vi "Search_Model.vi"(7 "LabVIEW Web Service Request":refnum<class "Web Request.lvclass">) -> (3 "html response":string)   [LabVIEW 2016]
uses:
  <vilib>/wsapi/Web Request.lvclass
  Device Info.ctl
  Inventory FGV Command.ctl
panel:
  # "Use the Web Service Request input terminal to call the VIs on the Web Services palette. Do not remove it from the connector pane unless you don't need access to the palette."
  # "Each additional control wired to the connector pane will be available as an input in the URL. To include an indicator in terminal-mode output (the default setting), it must also be wired to the connector pane."
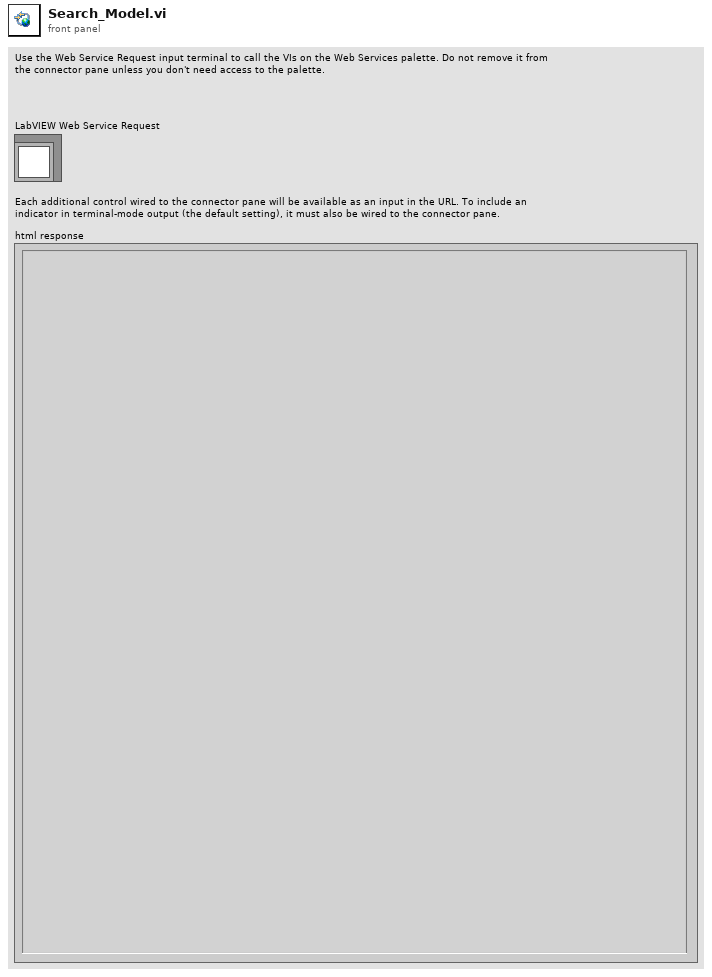
[diagram p1: front panel]
types:
  T1 = typedef "Inventory FGV Command.ctl" = enum16{"Load Items", "Check Status", "Return Items", "Check Out Items", "Add New Item", "Get All Items", "Remove Item", "Search"}
  T2 = typedef "Device Info.ctl" = cluster{"Model Number":string, "Identifier":string, "Available?":bool, "Owner":string, "Owner Email":string, "Last Activity Date":string, "Loan Purpose":string, "Department":string, "Notes":string, "Serial Number":string}
  T3 = typedef "Array Device Info.ctl" = T2[]
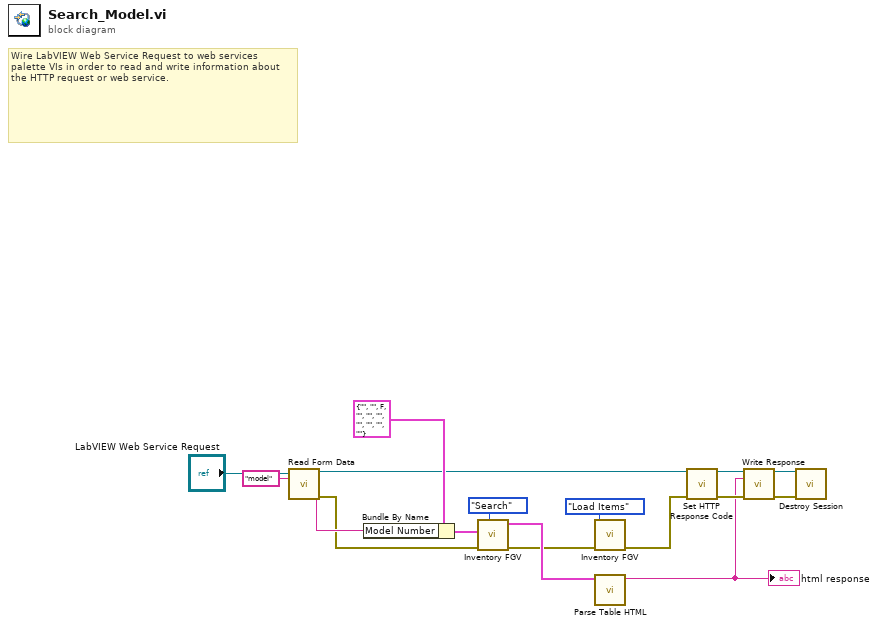
[diagram p0: block diagram]
diagram:
  # "Wire LabVIEW Web Service Request to web services palette VIs in order to read and write information about the HTTP request or web service."
  n1 = call <vilib>:"Read Form Data.vi"("LabVIEW Web Service Request"="LabVIEW Web Service Request", "key"="model") -> ("LabVIEW Web Service Request out"=w5:refnum<class "Web Request.lvclass">, "value"=w14:string, "error out"=w13:errorcluster)  [unwired: 10 in, 1 out]
  n2 = Bundle By Name(cluster=T2 {"Model Number"="", "Identifier"="", "Available?"=FALSE, "Owner"="", "Owner Email"="", "Last Activity Date"="", "Loan Purpose"="", "Department"="", "Notes"="", "Serial Number"=""} ("Device"), "Model Number"=w14) -> (w12:T2)
  n3 = call "Inventory FGV.vi"("error in"=w13, "Device Info"=w12, "Command"=Inventory_FGV_Command."Search") -> ("error out"=w3:errorcluster, "array of devices"=w10:T3)  [unwired: 5 in, 1 out]
  n4 = call "Inventory FGV.vi"("error in"=w3, "Command"=Inventory_FGV_Command."Load Items") -> ("error out"=w2:errorcluster)  [unwired: 6 in, 2 out]
  n5 = call "Parse Table HTML.vi"("array of devices"=w10) -> ("String"=w1:string)  [unwired: 10 in]
  "html response" <- w1
  n6 = call <vilib>:"Set HTTP Response Code.vi"("LabVIEW Web Service Request"=w5, "error in (no error)"=w2) -> ("LabVIEW Web Service Request out"=w9:refnum<class "Web Request.lvclass">, "error out"=w8:errorcluster)  [unwired: 12 in]
  n7 = call <vilib>:"Write Response.vi"("LabVIEW Web Service Request"=w9, "response string"=w1, "error in (no error)"=w8) -> ("LabVIEW Web Service Request out"=w7:refnum<class "Web Request.lvclass">, "error out"=w6:errorcluster)  [unwired: 11 in]
  n8 = call <vilib>:"Destroy Session.vi"("LabVIEW Web Service Request"=w7, "error in (no error)"=w6) -> ()  [unwired: 12 in, 2 out]
